vi "callback_recv_queue_obtain.vi"(8 "error in (no error)":errorcluster) -> (0 "error out":errorcluster, 3 "queue out":refnum<queue>)   [LabVIEW 2013, in "libssh2_integration_tests.lvlib"]
uses:
  libssh2_integration_tests.lvlib
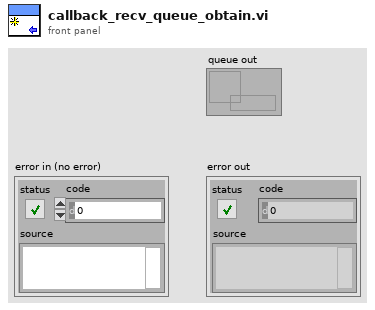
[diagram p1: front panel]
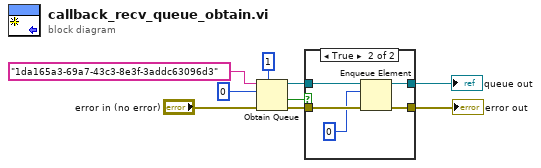
[diagram p0: block diagram]
diagram:
  n1 = Obtain Queue(max queue size (-1, unlimited)=1, name (unnamed)="1da165a3-69a7-43c3-8e3f-3addc63096d3", element data type=0, error in (no error)="error in (no error)") -> (queue out=w3:refnum<queue>, created new?=w1:bool, error out=w6:errorcluster)  [unwired: 1 in]
  n2 = case shown="True" w1 {
    tunnel: w6 -> [w10 w16]
    tunnel: [w10 w15] -> w4
    tunnel: w3 -> [w11 w14]
    tunnel: [w11 w13] -> w2
    frame False {
    }
    frame True {
      n3 = Enqueue Element(queue=w14, element=0, error in (no error)=w16) -> (queue out=w13:refnum<queue>, error out=w15:errorcluster)  [unwired: 1 in, 1 out]
    }
  }
  "error out" <- w4
  "queue out" <- w2
